vi "New_DetectionElectrodes.vi"() -> (2 "AreaName":string)   [LabVIEW 2014, in "DetectElectros.lvlib"]
uses:
  DetectElectros.lvlib
  <vilib>/Utility/file.llb/Read From Spreadsheet File (string).vi
  DataBase/DataBase.lvlib
panel:
  in  "导入电极s":path caption="导入数据"
  out "数组":string[](array[string])
  in  "OK":bool
  in  "退出":bool
  in  "提交数据":bool
  in  "导入电极":bool
  in  "电极管理_新增":string[][](table)
  in  "电极管理_新增列表":i32[](listbox)
  in  "区域名称":u16(ring) items=["1区", "2区"]
  out "error out":errorcluster caption="错误输出"
  in  "error in (no error)":errorcluster caption="错误输入（无错误）"
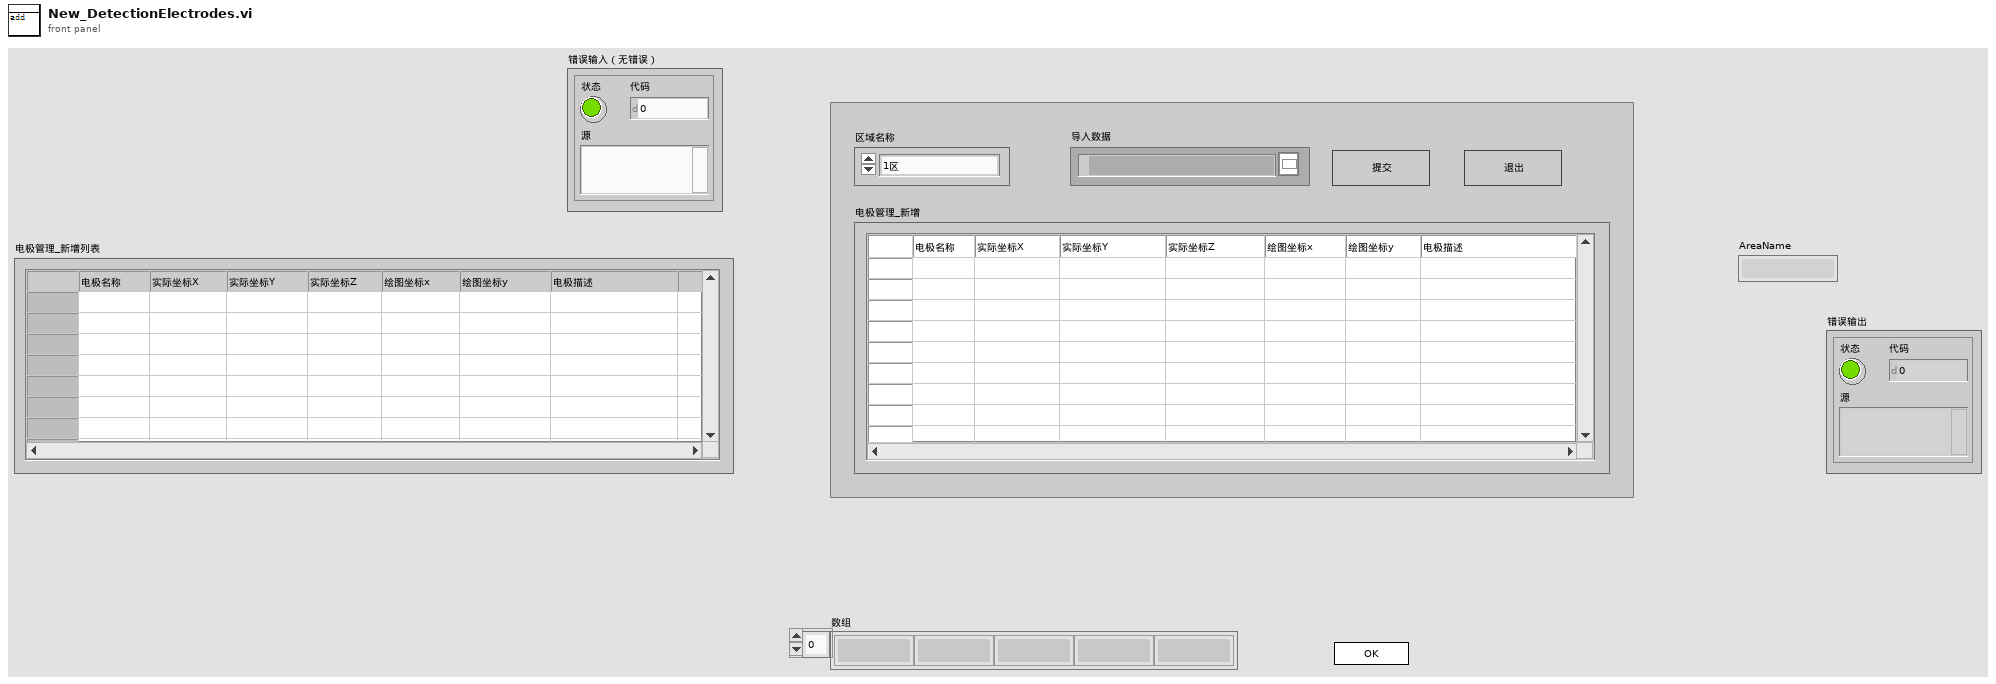
[diagram p1: front panel]
types:
  T1 = enum32{"invalid app kind", "Development System", "Run Time System", "Student Edition", "Embedded LabVIEW", "Evaluation", "Custom"}
  T2 = enum32{"Invalid", "Standard", "Closed", "Hidden", "Minimized", "Maximized"}
  T3 = cluster{"Core":cluster{"Current VI Reference":refnum<vi>, "Close Panel on Exit?":bool}, "Your Boolean data":bool, "Your string data":string, "AreaNameD":string}
  T4 = cluster{"Current VI Reference":refnum<vi>, "Close Panel on Exit?":bool}
  T5 = cluster{"String":string, "String":string, "String":string, "String":string, "String":string, "String":string, "String":string, "String":string, "String":string, "String":string, "String":string, "String":string}
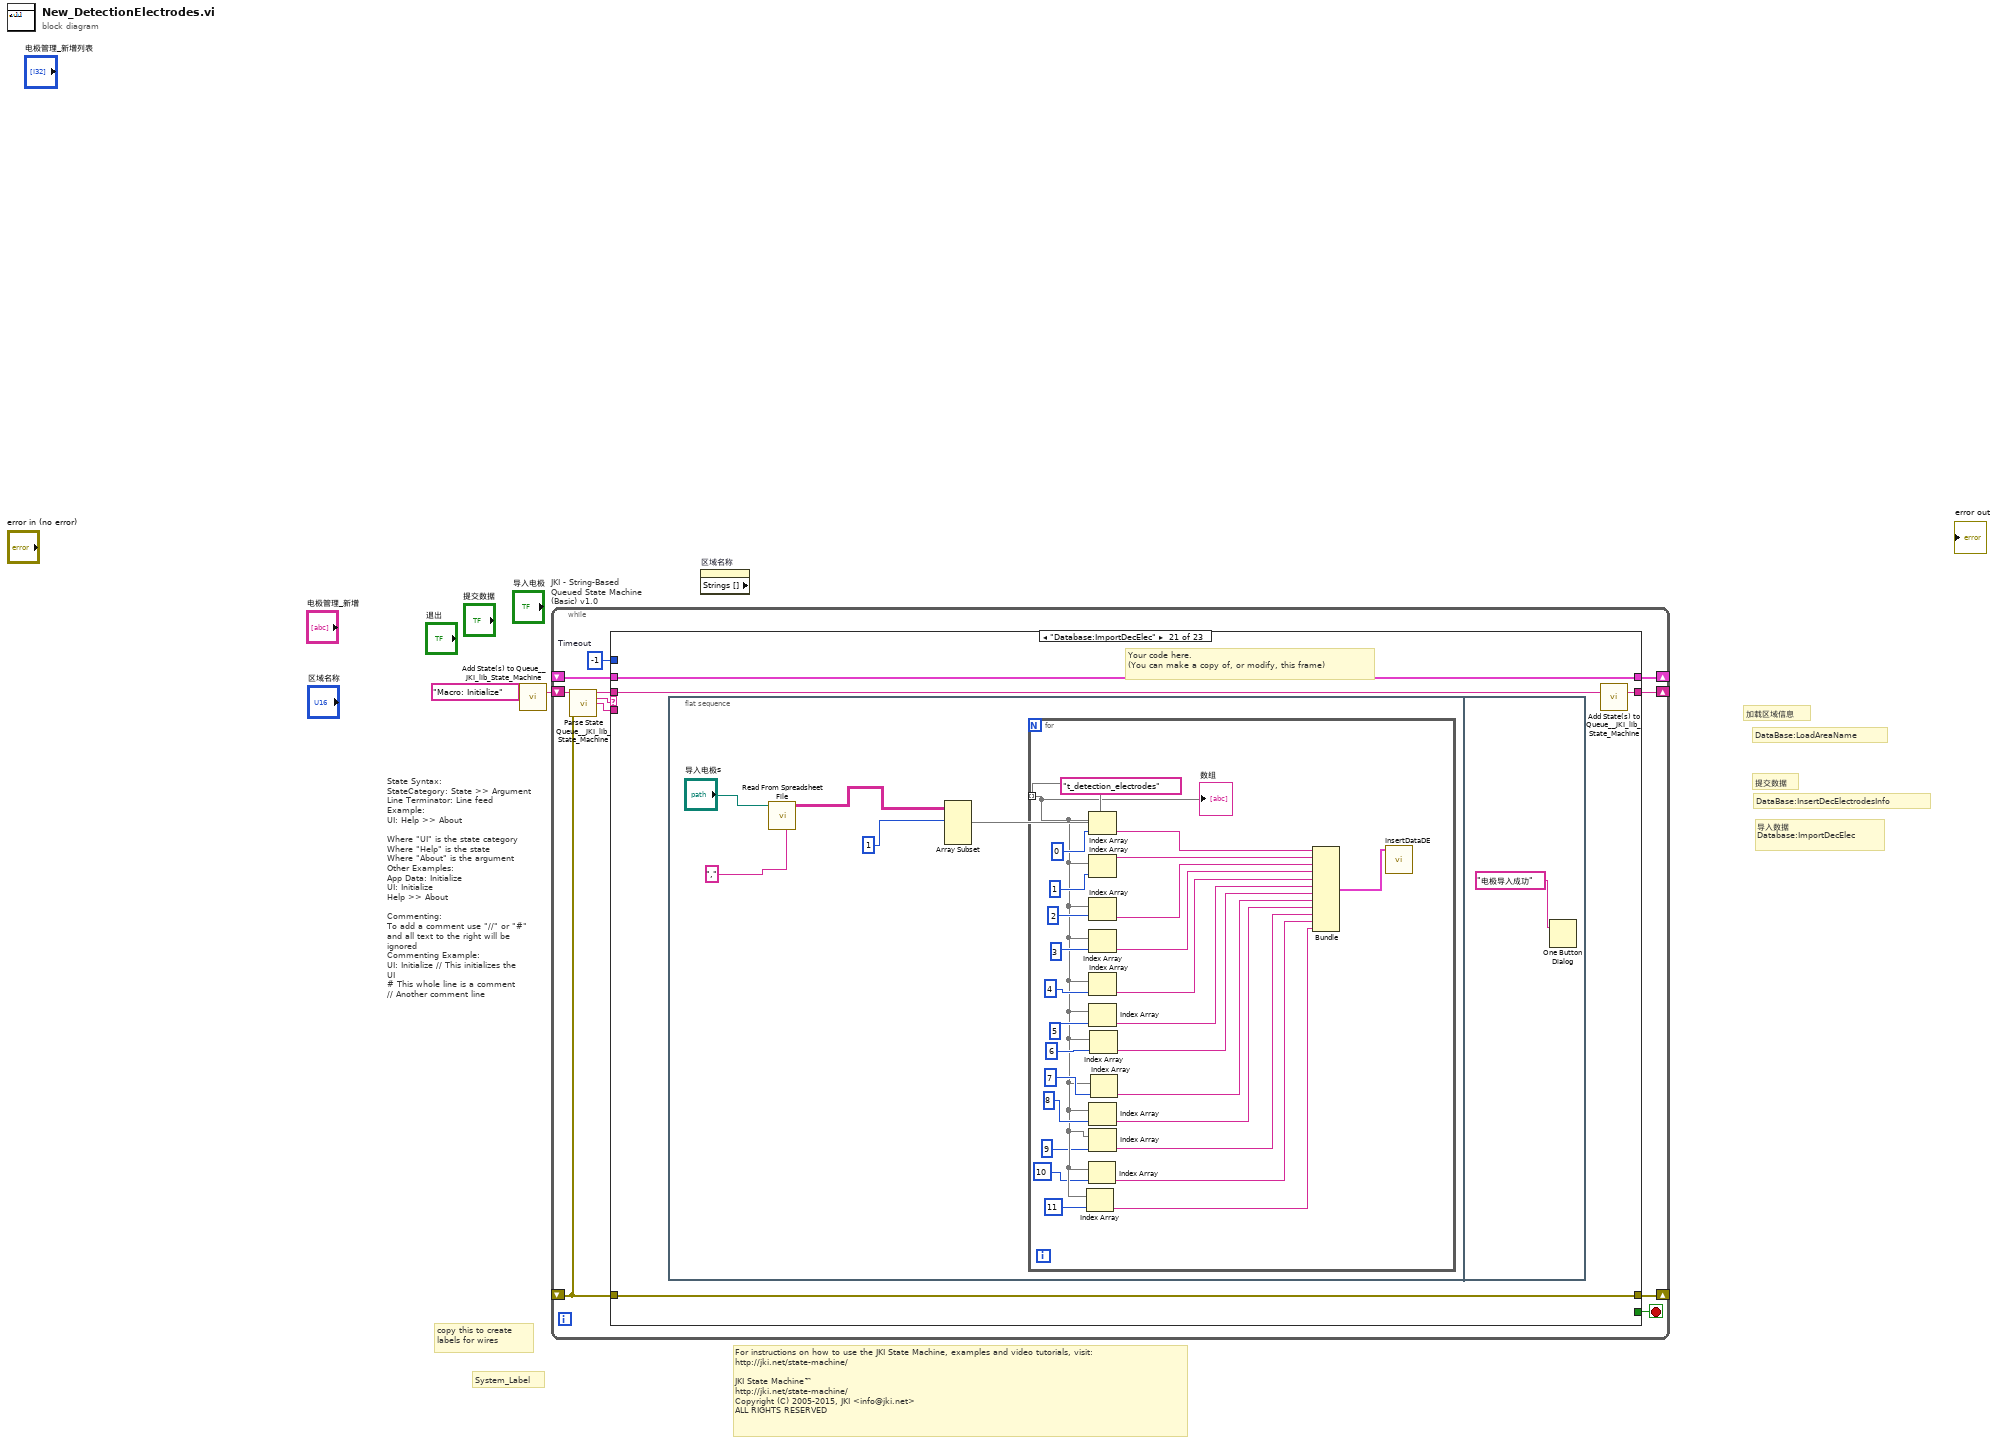
[diagram p0: block diagram]
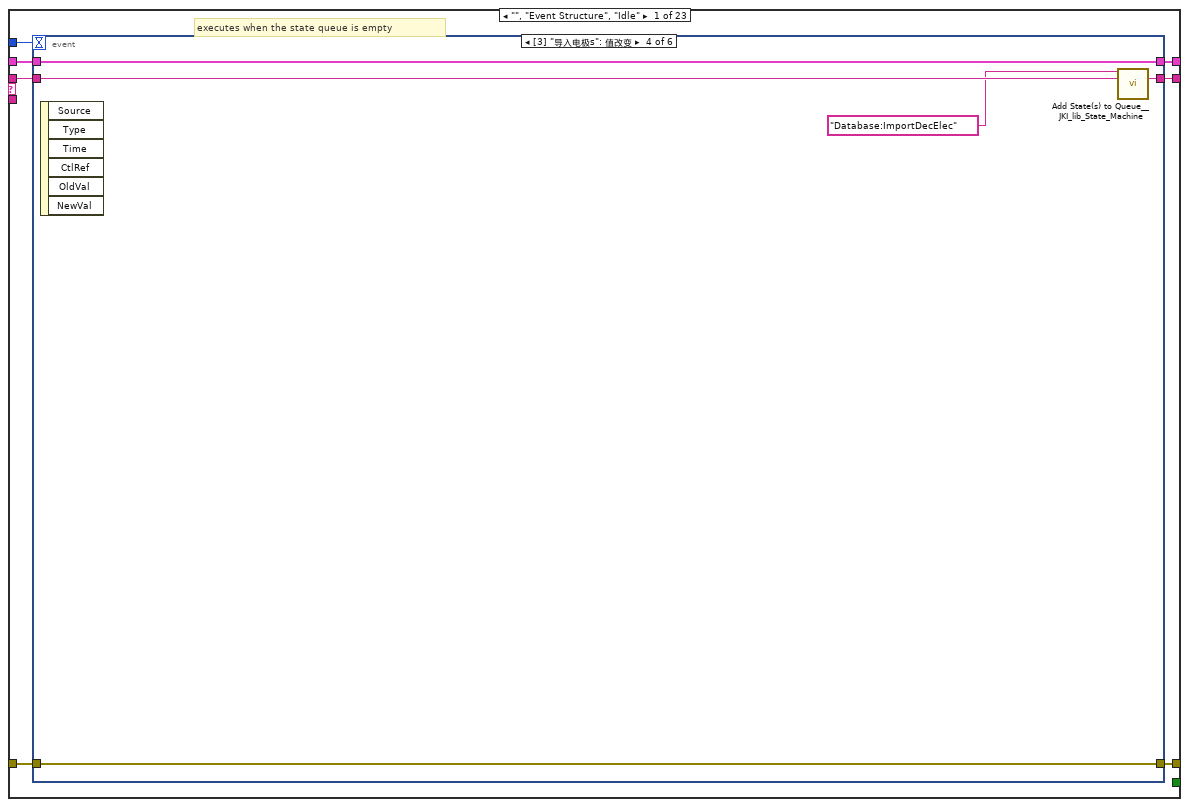
[diagram p2: hidden frame]
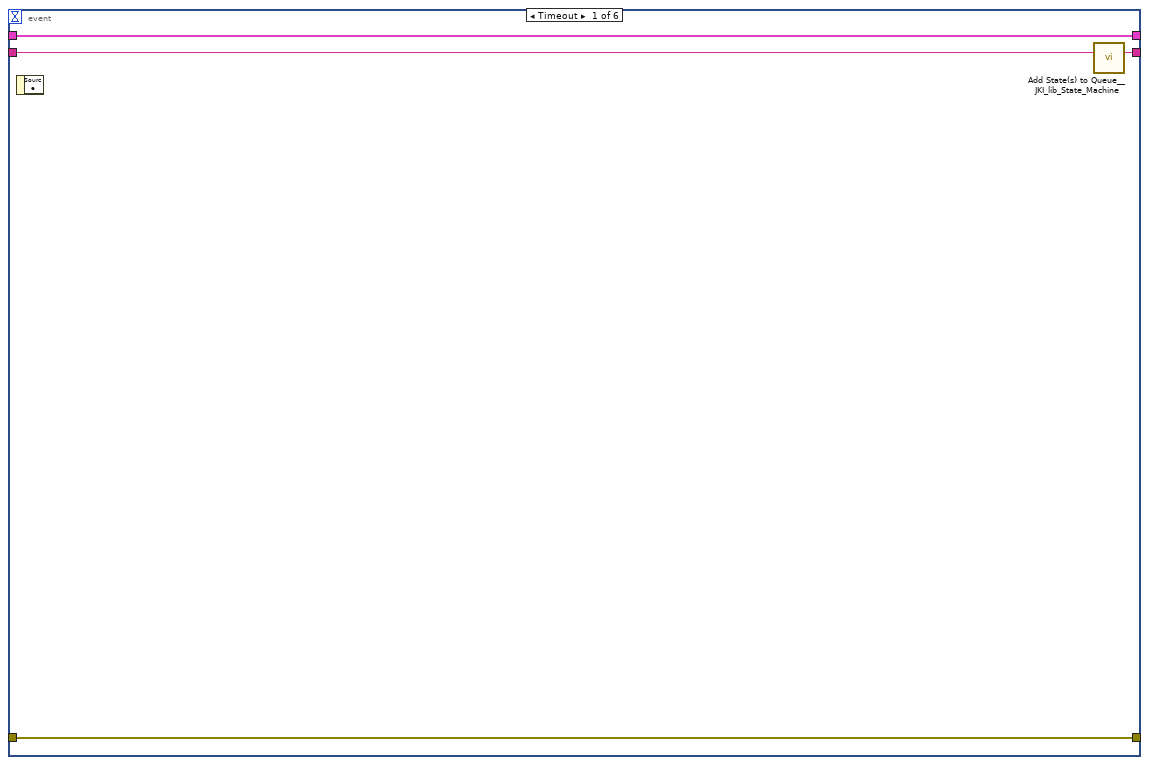
[diagram p3: hidden frame]
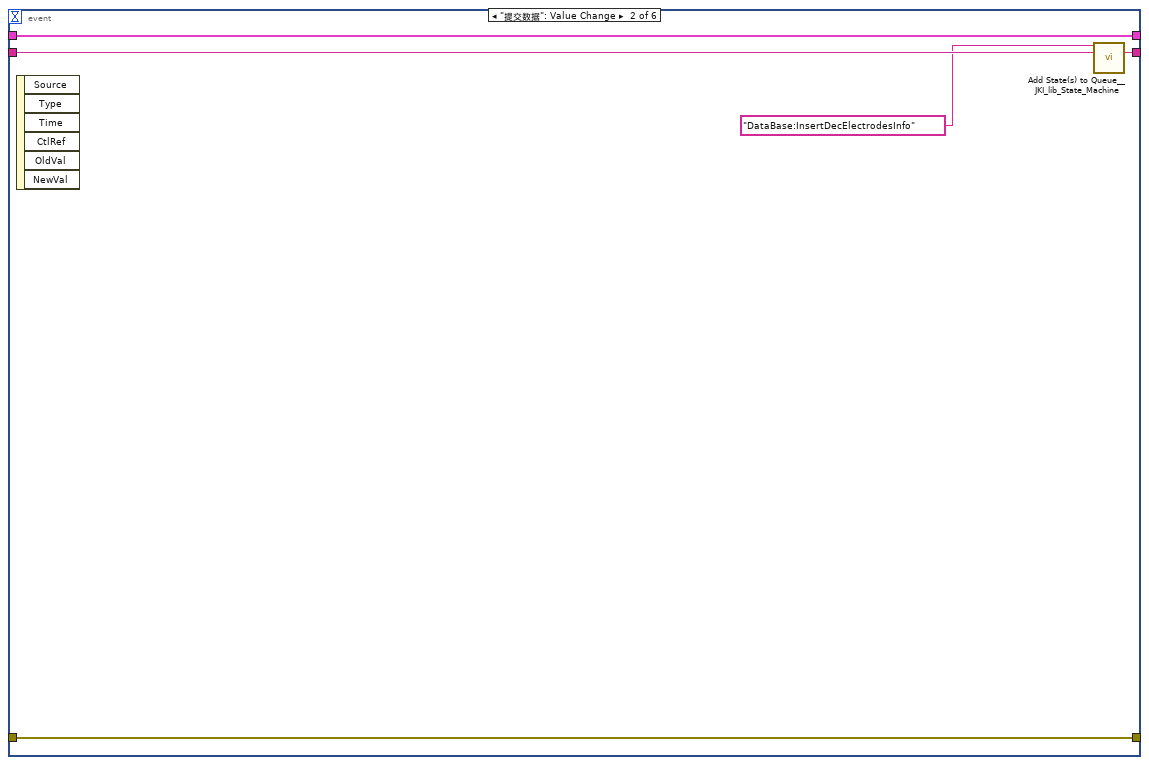
[diagram p4: hidden frame]
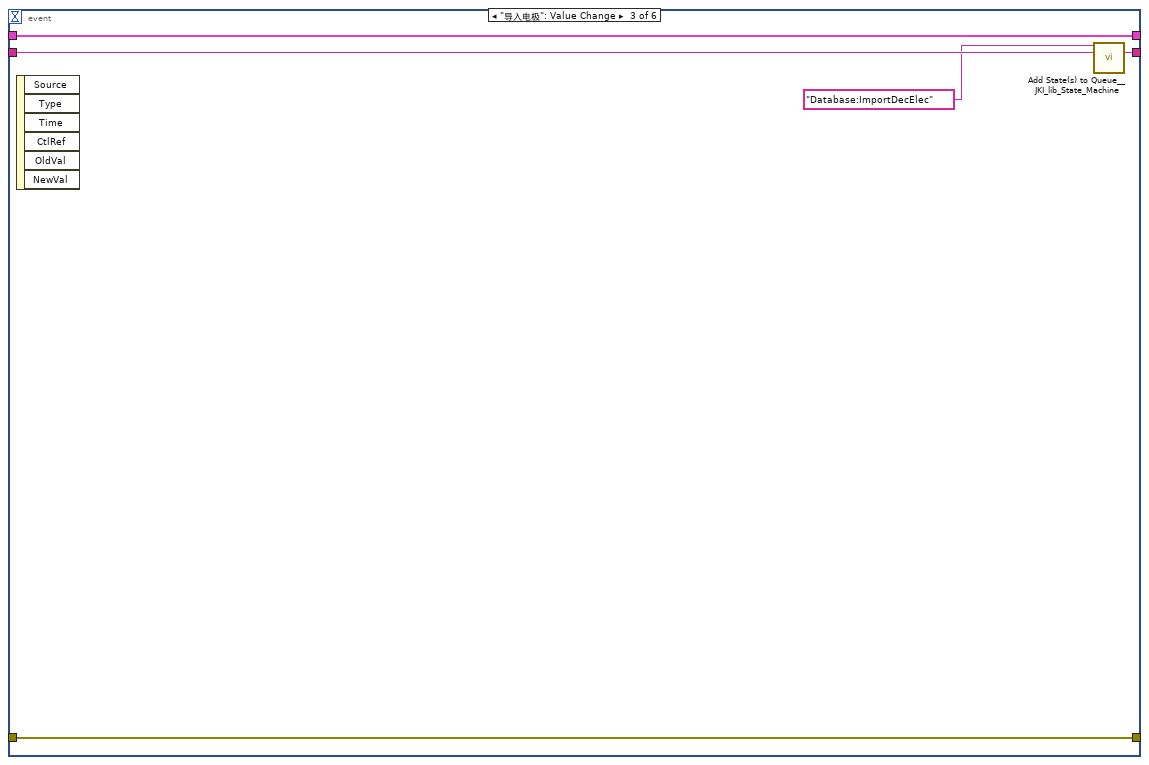
[diagram p5: hidden frame]
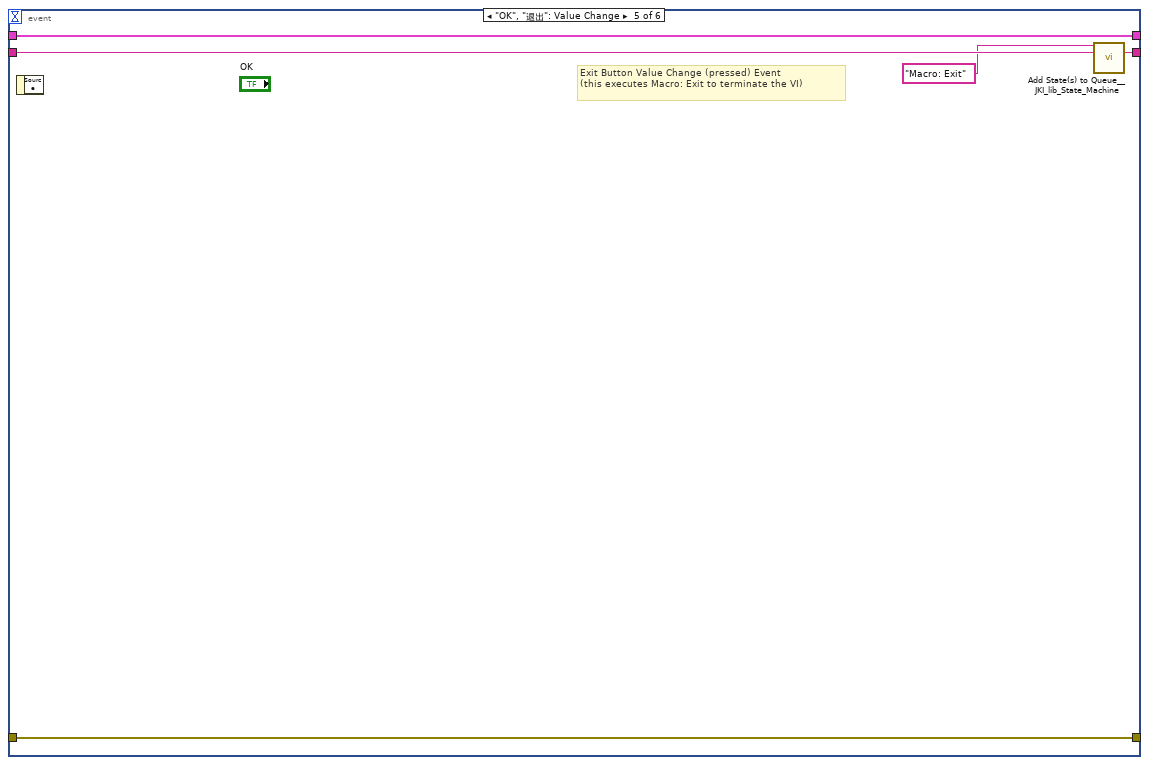
[diagram p6: hidden frame]
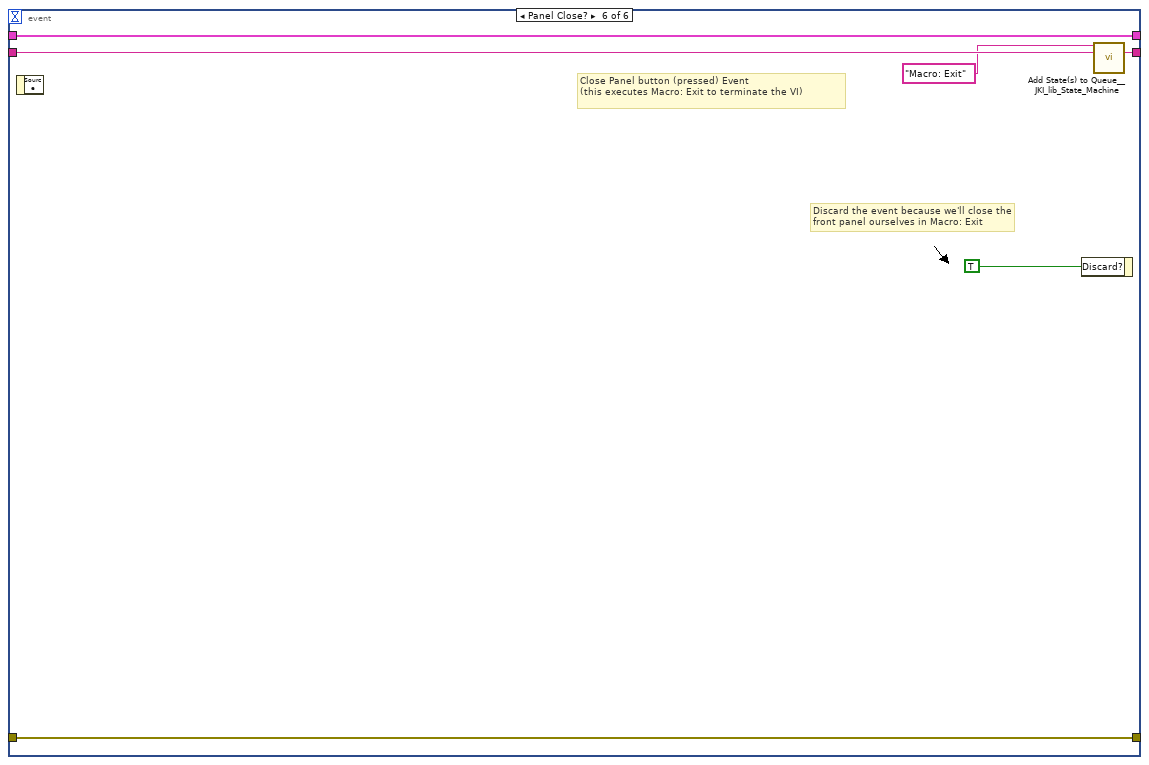
[diagram p7: hidden frame]
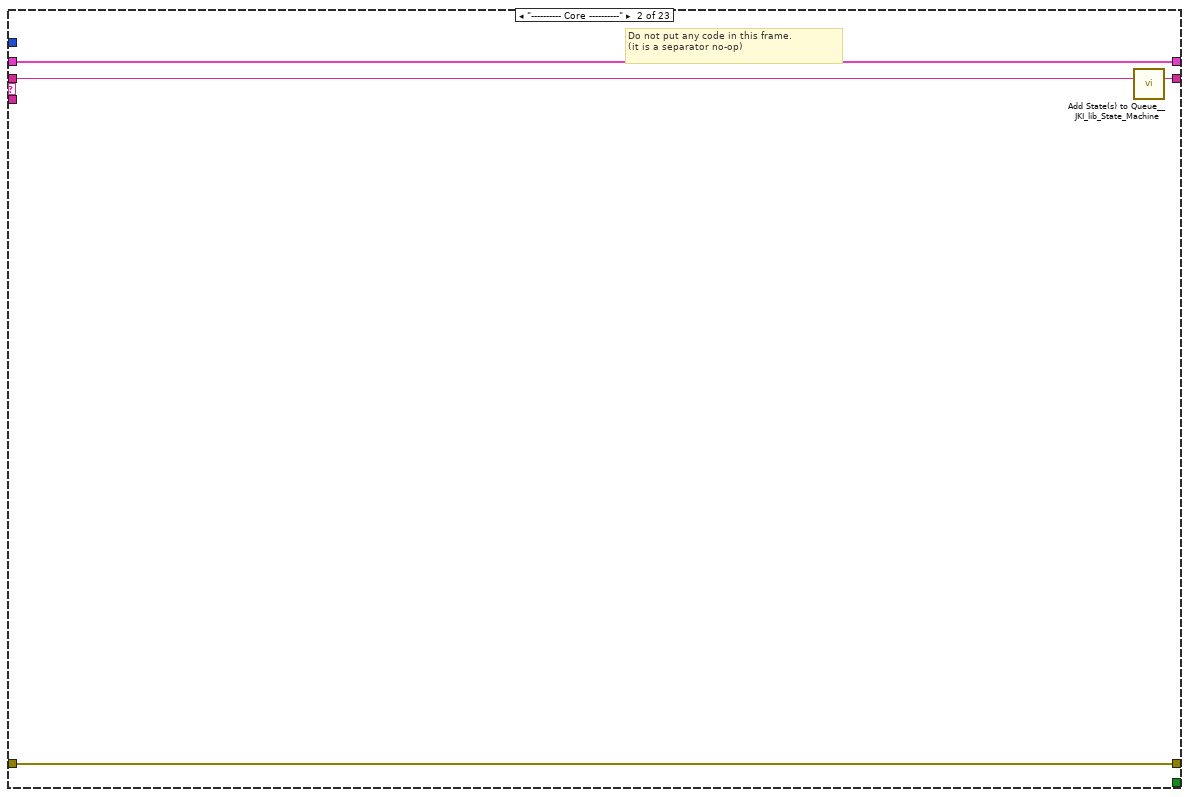
[diagram p8: hidden frame]
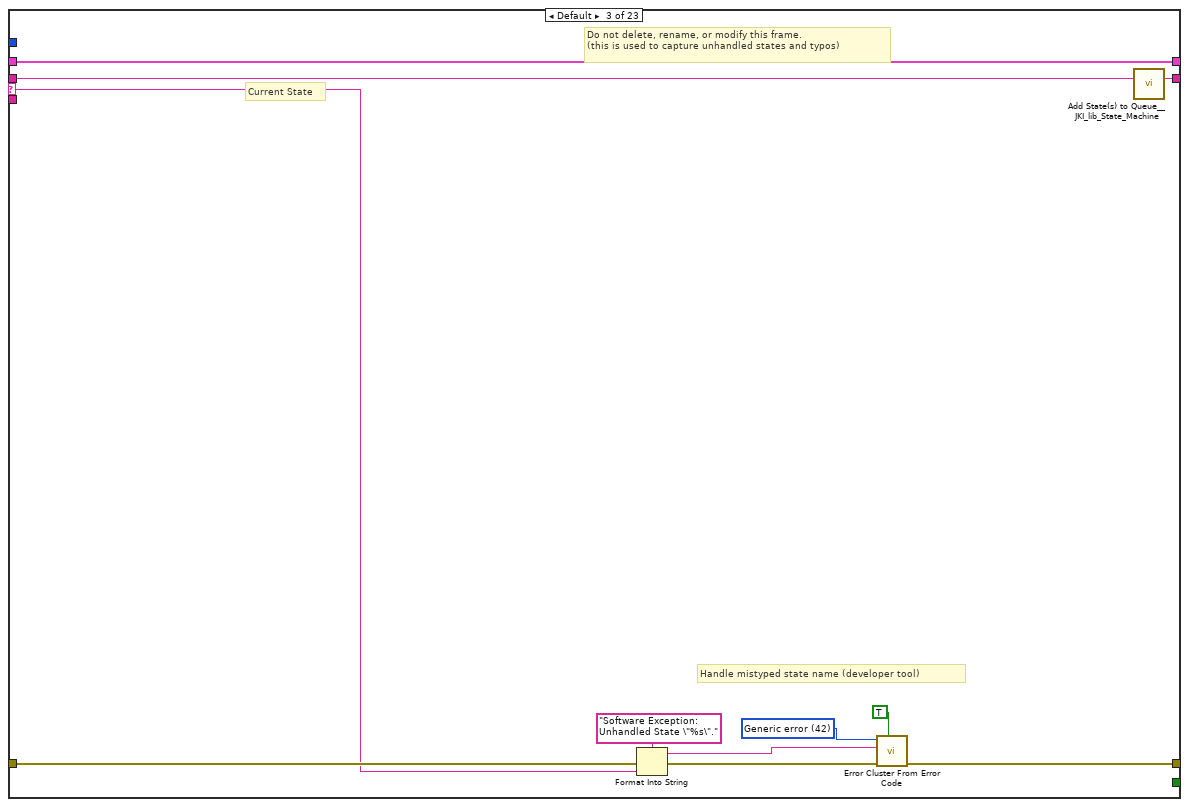
[diagram p9: hidden frame]
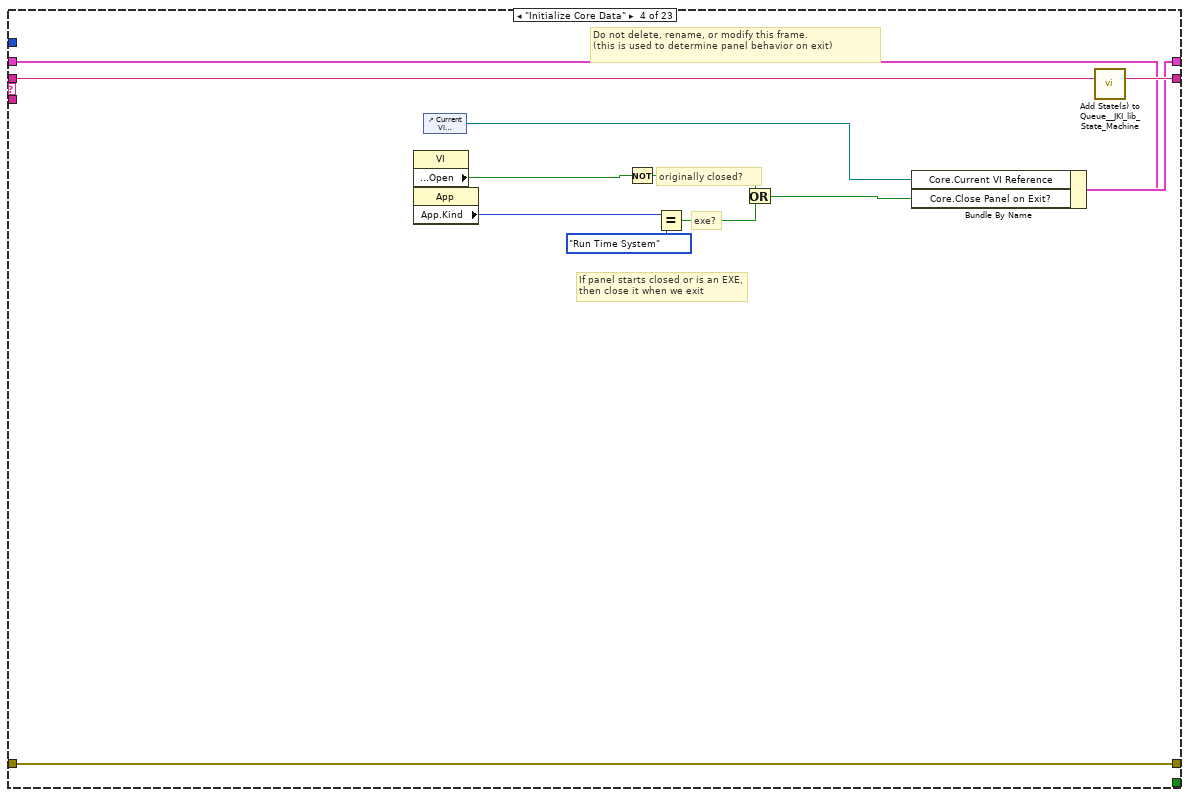
[diagram p10: hidden frame]
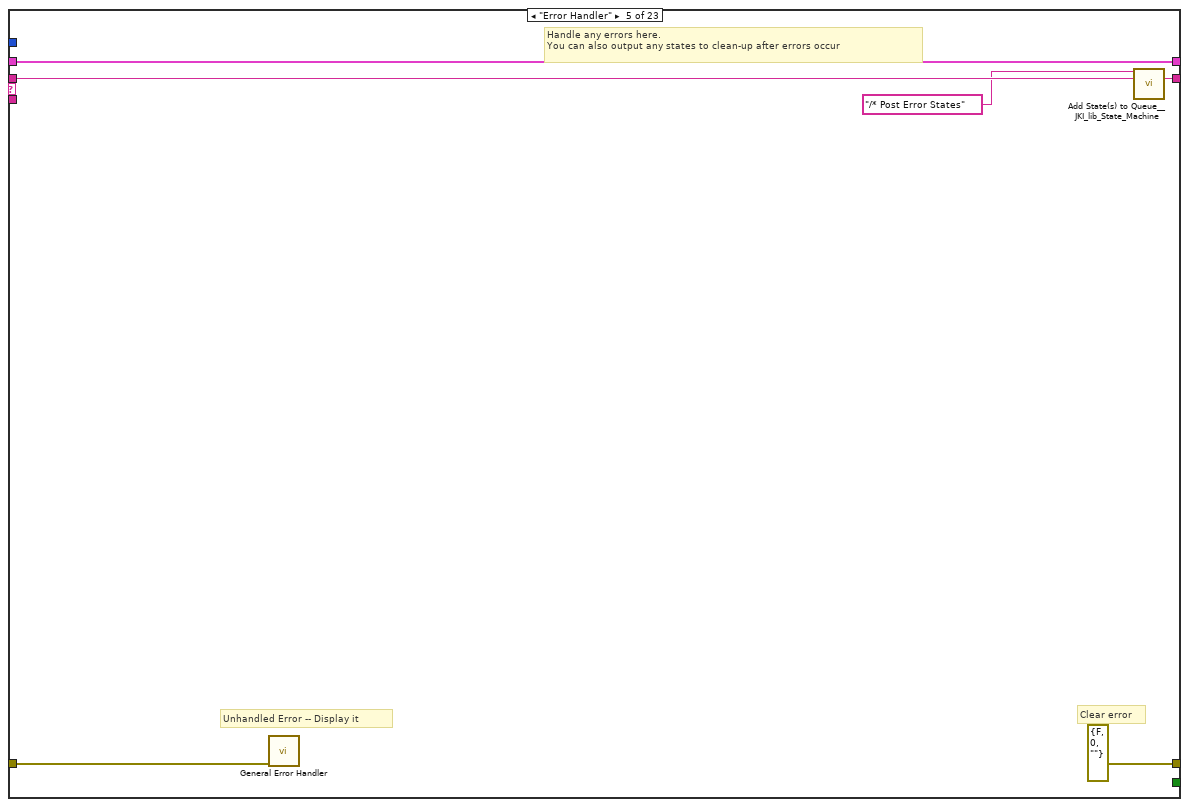
[diagram p11: hidden frame]
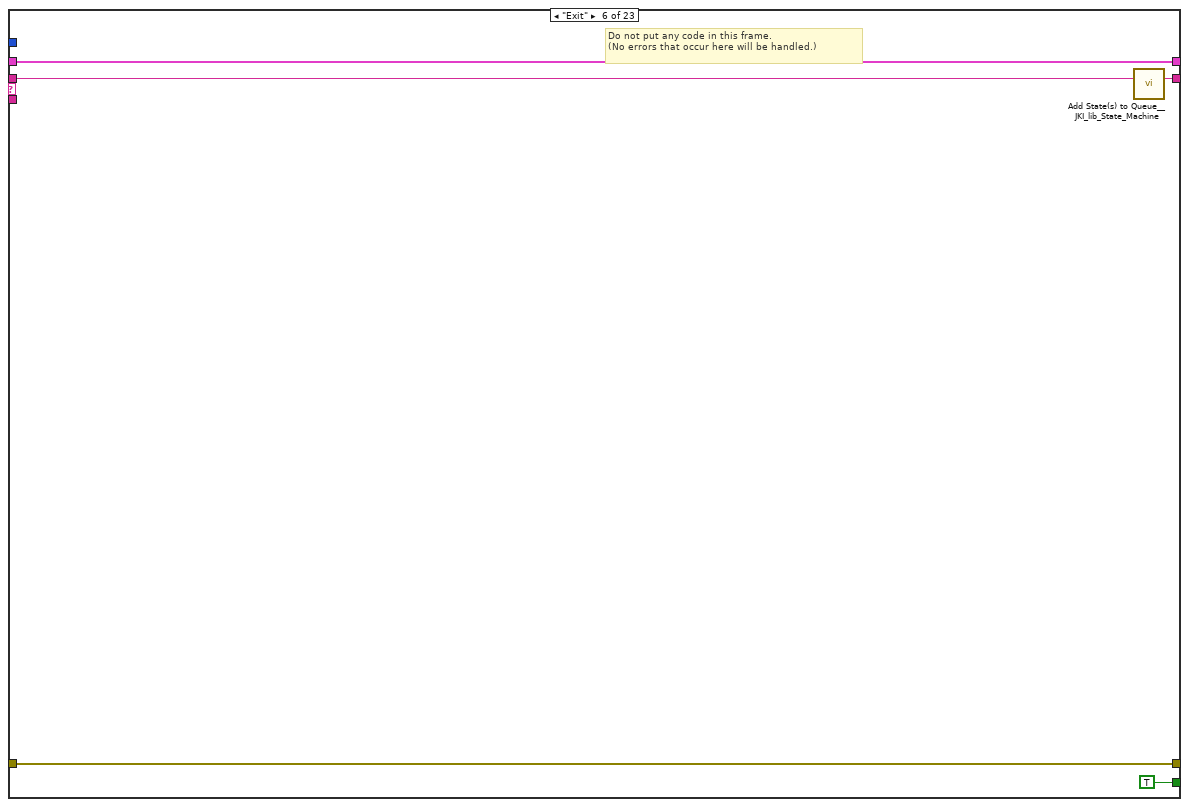
[diagram p12: hidden frame]
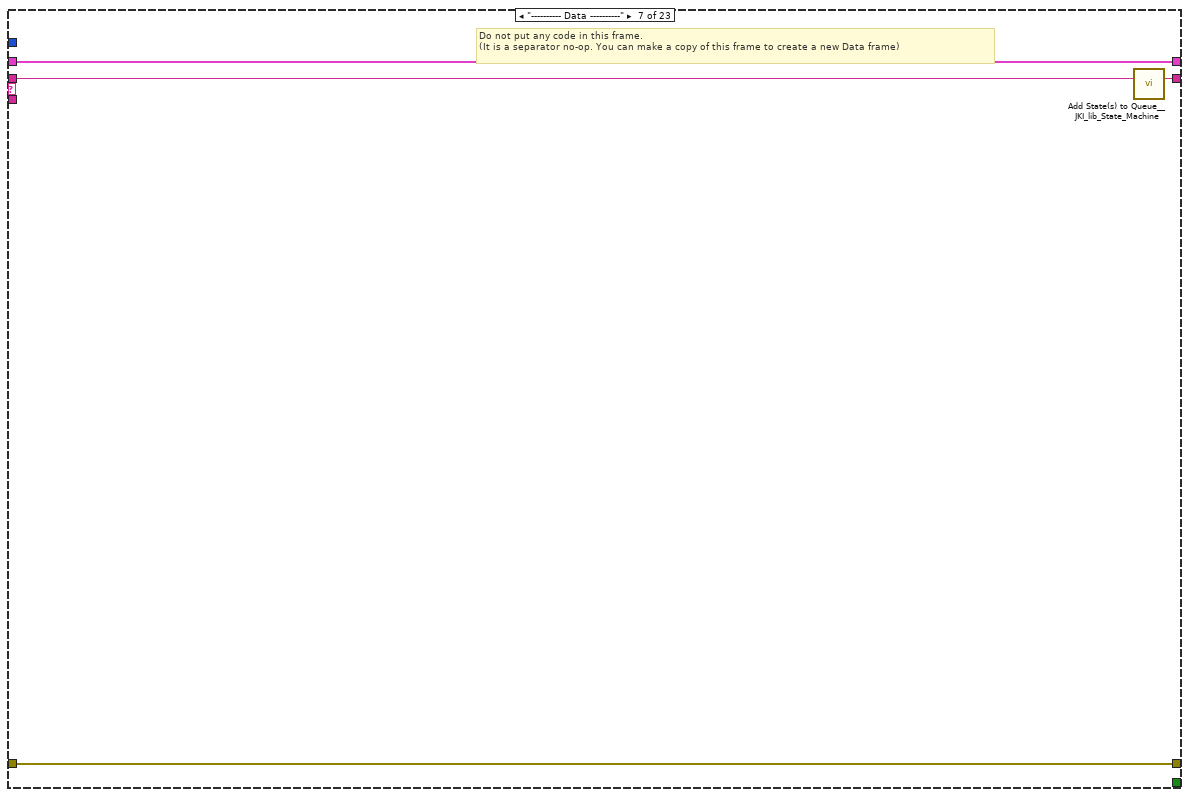
[diagram p13: hidden frame]
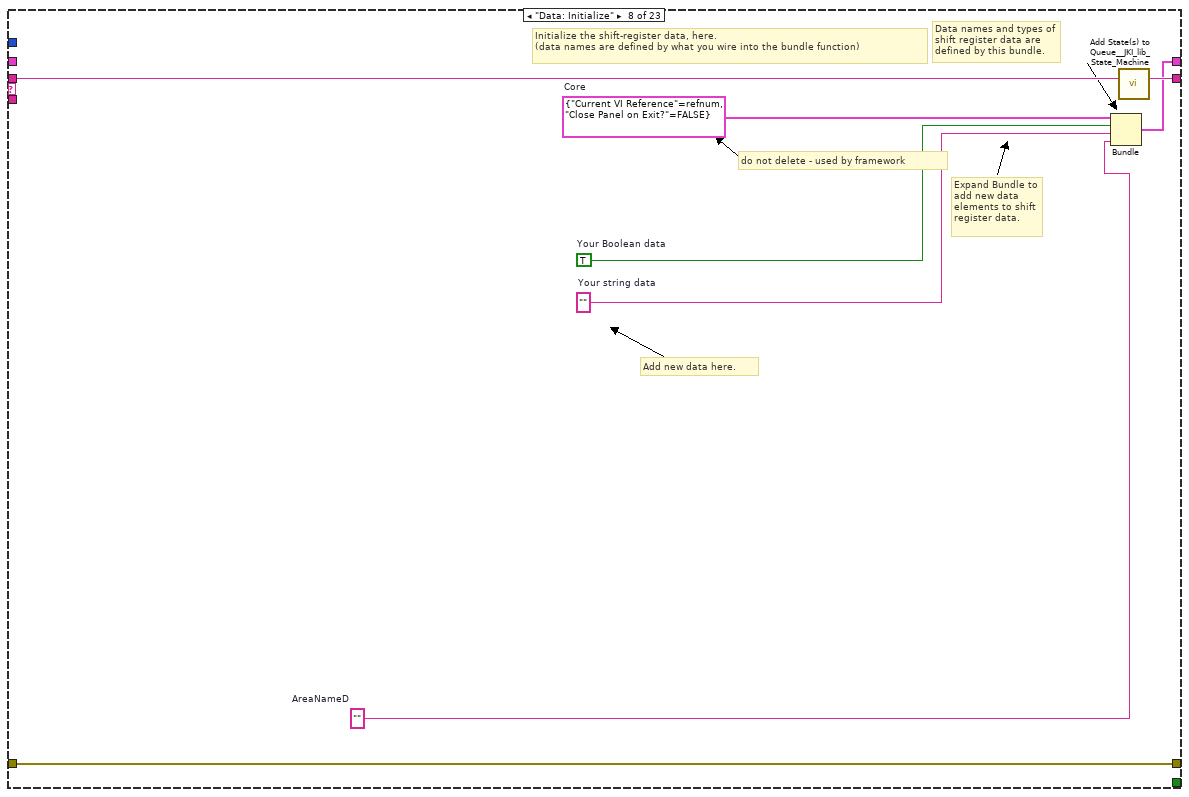
[diagram p14: hidden frame]
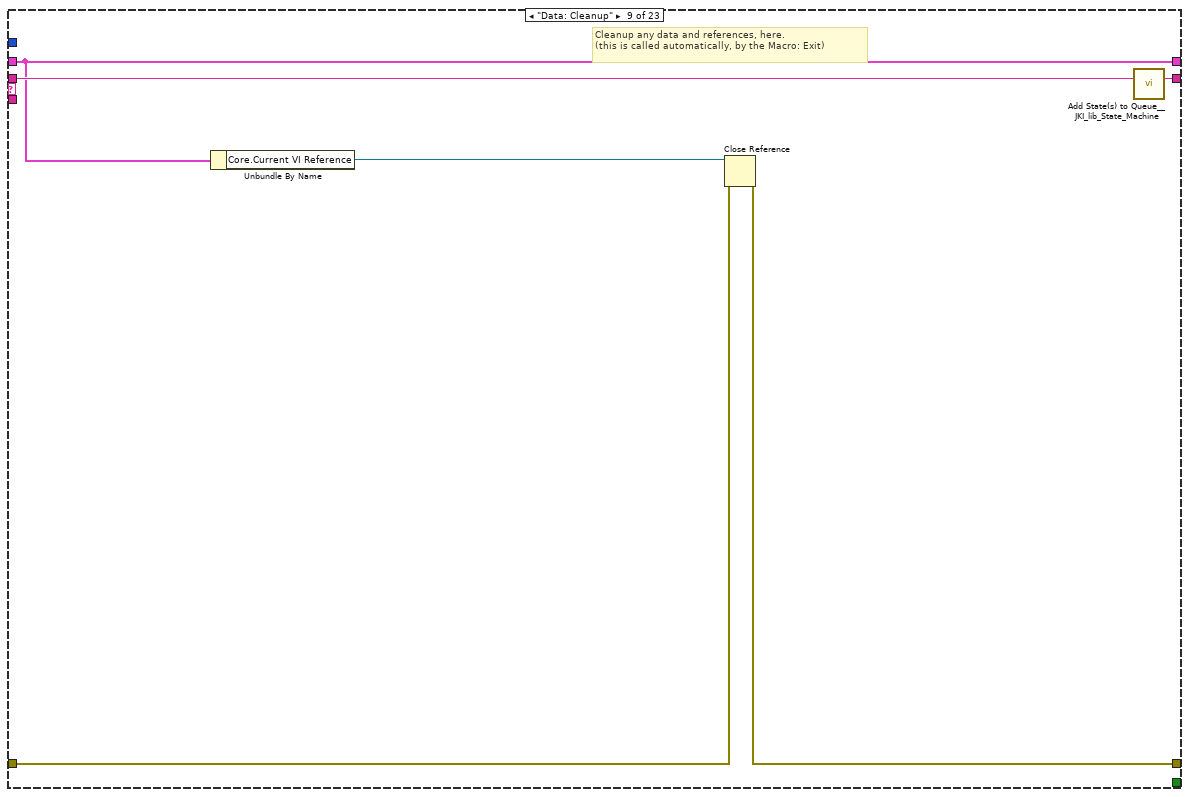
[diagram p15: hidden frame]
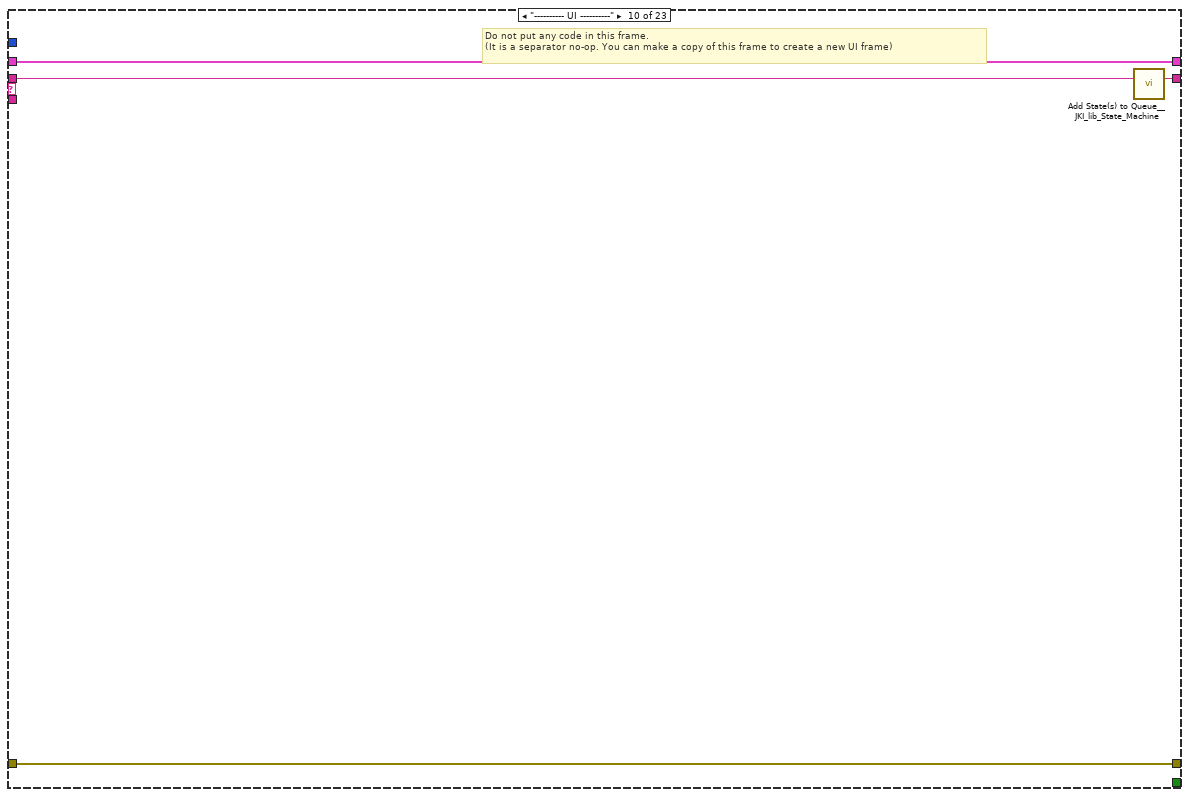
[diagram p16: hidden frame]
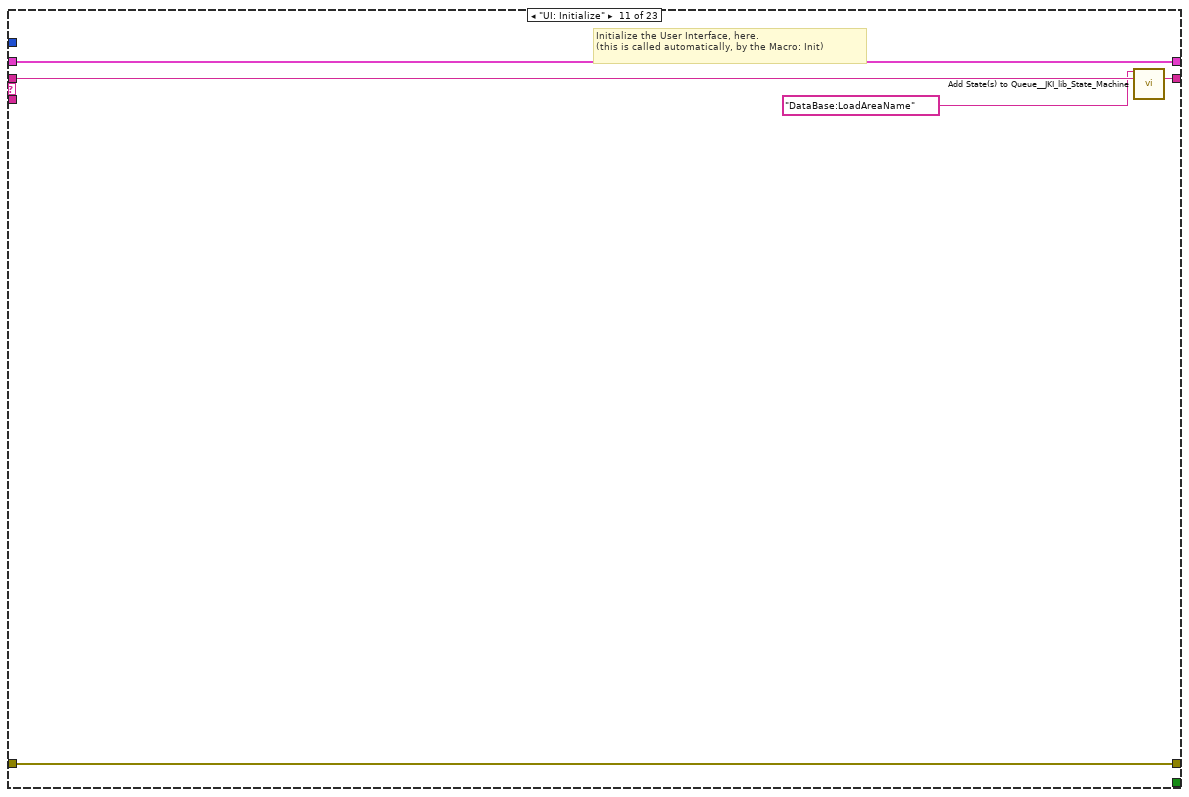
[diagram p17: hidden frame]
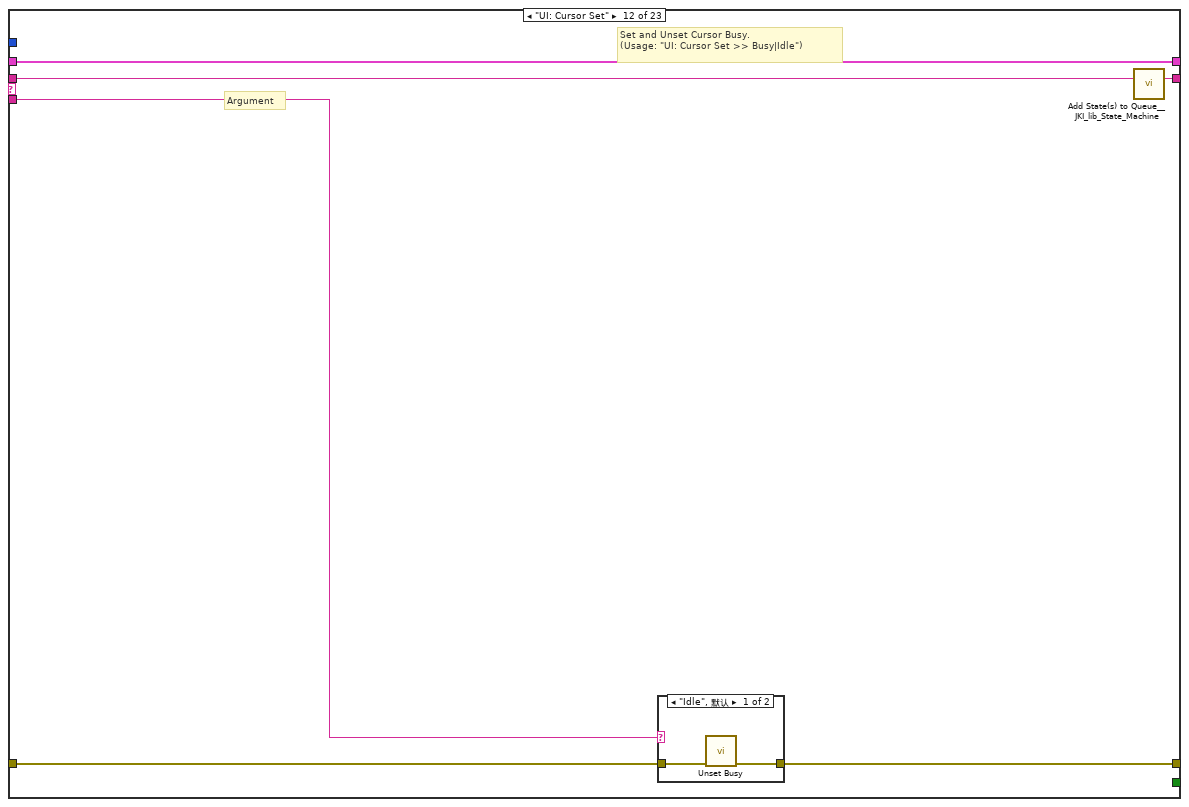
[diagram p18: hidden frame]
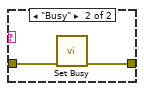
[diagram p19: hidden frame]
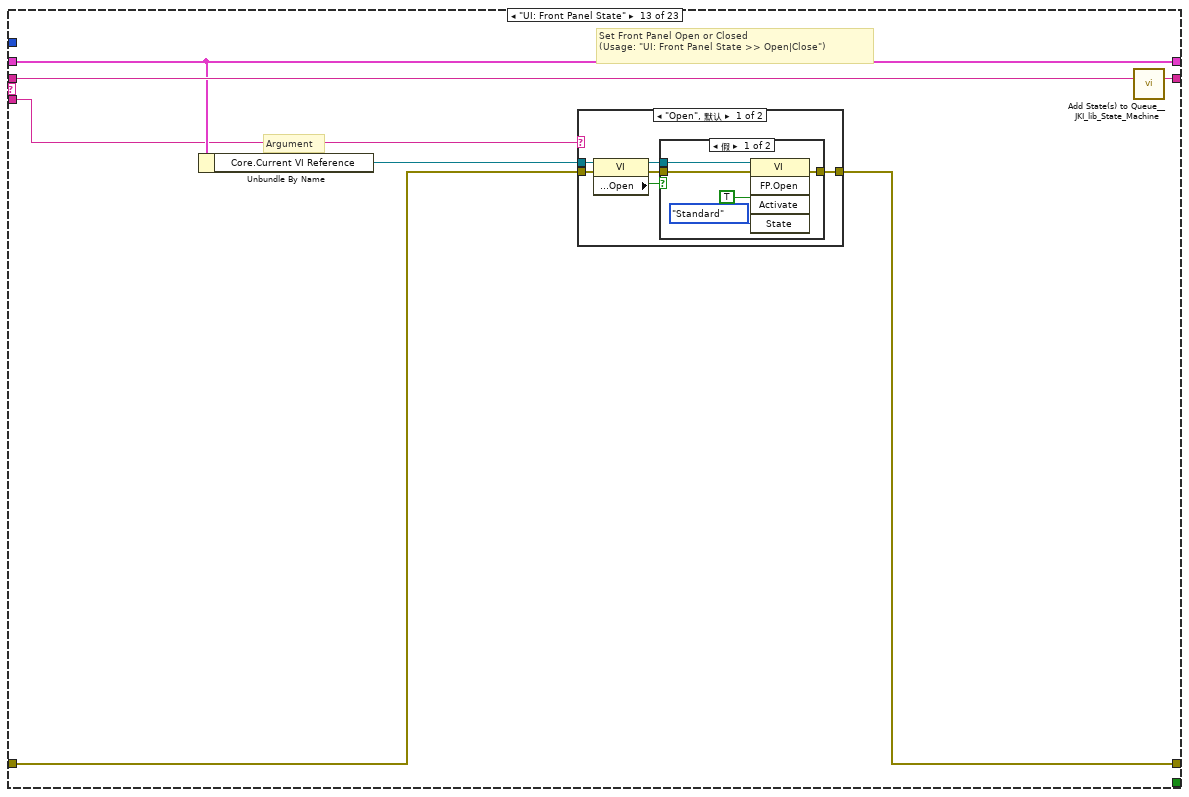
[diagram p20: hidden frame]
diagram:
  # "导入数据\nDatabase:ImportDecElec"
  # "DataBase:InsertDecElectrodesInfo"
  # "提交数据"
  # "DataBase:LoadAreaName"
  # "加载区域信息"
  # "For instructions on how to use the JKI State Machine, examples and video tutorials, visit:\nhttp://jki.net/state-machine/\n\nJKI State Machine™\nhttp://jki.net/state-machine/\nCopyright (C) 2005-2015, JKI <info@jki.net>\nALL RIGHTS RESERVED"
  # "State Syntax:\nStateCategory: State >> Argument\nLine Terminator: Line feed\nExample:\nUI: Help >> About\n\nWhere \"UI\" is the state category\nWhere \"Help\" is the state\nWhere \"About\" is the argument\nOther Examples:\nApp Data: Initialize\nUI: Initialize\nHelp >> About\n\nCommenting:\nTo add a comment use \"//\" or \"#\" and all text to the right will be ignored\nCommenting Example:\nUI: Initialize // This initializes the UI\n# This whole line is a comment\n// Another comment line"
  # "copy this to create labels for wires"
  # "System_Label"
  n1 = call <vilib>:"Add State(s) to Queue__JKI_lib_State_Machine.vi"("State(s) in (\"\")"="Macro: Initialize") -> ("States Out"=w2:string)  [unwired: 14 in]
  n2 = while "JKI - String-Based Queued State Machine (Basic) v1.0" {
    shift-right: [w6] -> _
    shift-left: _ -> [w5]
    shift-right: [w9] -> _
    shift-left: _ -> [w3]
    shift-right: [w8] -> _
    shift-left: w2 -> [w10]
    stop <- w7 stop-if-true
    w4 = -1  # Timeout
    n3 = call <vilib>:"Parse State Queue__JKI_lib_State_Machine.vi"("State Queue"=w10, "Error In (no error)"=w3) -> ("Remaining States"=w12:string, "Current State"=w13:string, "Arguments"=w11:string)  [unwired: 11 in]
    n4 = case shown="\"Database:ImportDecElec\"" w13 {
      selector: w13 -> [_ _ w55 _ _ _ _ _ _ _ _ _ _ _ _ _ _ _ _ _ _ _ _]
      tunnel: w12 -> [w20 w54 w59 w77 w83 w88 w92 w100 w106 w110 w115 w121 w132 w158 w163 w173 w177 w181 w185 w189 w193 w233 w259]
      tunnel: w11 -> [_ _ _ _ _ _ _ _ _ _ _ w116 w126 _ _ _ _ _ _ _ _ _ _]
      tunnel: w5 -> [w18 w51 w57 w68 w80 w86 w89 _ w101 w107 w113 w119 w128 w155 w160 w170 w174 w178 w182 w186 w190 w226 w247]
      tunnel: [w17 w52 w61 w74 errorcluster {"status"=FALSE, "code"=0, "source"=""} ("error out") w85 w90 w97 w102 w108 w112 w117 w129 w156 w161 w171 w175 w179 w183 w187 w191 w227 w251] -> w9
      tunnel: w3 -> [w16 w52 w60 w74 w79 w85 w90 w97 w103 w108 w112 w118 w130 w156 w161 w171 w175 w179 w183 w187 w191 w228 w251]
      tunnel: [w19 w53 w58 w76 w82 w87 w91 w99 w105 w109 w114 w120 w131 w157 w162 w172 w176 w180 w184 w188 w192 w232 w258] -> w8
      tunnel: [_ _ _ _ _ TRUE _ _ _ _ _ _ _ _ _ _ _ _ _ _ _ _ _] -> w7
      tunnel: [w15 w51 w57 w75 w80 w86 w89 w98 w101 w107 w113 w119 w128 w155 w160 w170 w174 w178 w182 w186 w190 w226 w246] -> w6
      tunnel: w4 -> [w14 _ _ _ _ _ _ _ _ _ _ _ _ _ _ _ _ _ _ _ _ _ _]
      frame "", "Event Structure", "Idle" {
        # "executes when the state queue is empty"
        n5 = event shown="[3] \"导入电极s\": 值改变" {
          selector: _ -> [_ _ _ _ _ _]
          dyn-events: _ -> [_ _ _ _ _ _]
          timeout: w14 -> [_ _ _ _ _ _]
          tunnel: w20 -> [w24 w29 w34 w39 w44 w50]
          tunnel: [w23 w28 w33 w38 w43 w49] -> w19
          tunnel: w18 -> [w21 w26 w31 w36 w41 w47]
          tunnel: [w22 w27 w32 w37 w42 w48] -> w17
          tunnel: w16 -> [w22 w27 w32 w37 w42 w48]
          tunnel: [w21 w26 w31 w36 w41 w47] -> w15
          event Timeout {
            n6 = event-data() -> ()  [unwired: 1 in, 1 out]
            n7 = call <vilib>:"Add State(s) to Queue__JKI_lib_State_Machine.vi"("State(s) in (\"\")"=w24) -> ("States Out"=w23:string)  [unwired: 14 in]
          }
          event "提交数据": Value Change {
            n8 = event-data() -> ()  [unwired: 1 in, 6 out]
            n9 = call <vilib>:"Add State(s) to Queue__JKI_lib_State_Machine.vi"("State(s) in Front (\"\")"="DataBase:InsertDecElectrodesInfo", "State(s) in (\"\")"=w29) -> ("States Out"=w28:string)  [unwired: 13 in]
          }
          event "导入电极": Value Change {
            n10 = event-data() -> ()  [unwired: 1 in, 6 out]
            n11 = call <vilib>:"Add State(s) to Queue__JKI_lib_State_Machine.vi"("State(s) in Front (\"\")"="Database:ImportDecElec", "State(s) in (\"\")"=w34) -> ("States Out"=w33:string)  [unwired: 13 in]
          }
          event "导入电极s": Value Change {
            n12 = event-data() -> ()  [unwired: 1 in, 6 out]
            n13 = call <vilib>:"Add State(s) to Queue__JKI_lib_State_Machine.vi"("State(s) in Front (\"\")"="Database:ImportDecElec", "State(s) in (\"\")"=w39) -> ("States Out"=w38:string)  [unwired: 13 in]
          }
          event "OK", "退出": Value Change {
            # "Exit Button Value Change (pressed) Event\n(this executes Macro: Exit to terminate the VI)"
            n14 = event-data() -> ()  [unwired: 1 in, 1 out]
            n15 = call <vilib>:"Add State(s) to Queue__JKI_lib_State_Machine.vi"("State(s) in Front (\"\")"="Macro: Exit", "State(s) in (\"\")"=w44) -> ("States Out"=w43:string)  [unwired: 13 in]
          }
          event Panel Close? {
            # "Discard the event because we'll close the front panel ourselves in Macro: Exit"
            # "Close Panel button (pressed) Event\n(this executes Macro: Exit to terminate the VI)"
            n16 = event-data() -> ()  [unwired: 1 in, 1 out]
            n17 = event-data("Discard?"=TRUE) -> ()  [unwired: 1 in, 1 out]
            n18 = call <vilib>:"Add State(s) to Queue__JKI_lib_State_Machine.vi"("State(s) in Front (\"\")"="Macro: Exit", "State(s) in (\"\")"=w50) -> ("States Out"=w49:string)  [unwired: 13 in]
          }
        }
      }
      frame "---------- Core ----------" {
        # "Do not put any code in this frame.\n(it is a separator no-op)"
        n19 = call <vilib>:"Add State(s) to Queue__JKI_lib_State_Machine.vi"("State(s) in (\"\")"=w54) -> ("States Out"=w53:string)  [unwired: 14 in]
      }
      frame Default {
        w64 = 42 items=["No error", "Argument error", "Memory is full", "Out of zone", "End of file", "File already open", "Generic file I/O error", "File not found", "File permission error", "Disk is full", "Duplicate path", "Too many files open", "System feature not enabled", "Resource file not found", "Cannot add resource", "Resource not found", "Image not found", "Image memory error", "Pen does not exist", "Config type invalid", "Config token not found", "Config parse error", "Config memory error", "Bad external code format", "Bad external code offset", "External code not present", "Null window", "Destroy window error", "Null menu", "Print aborted", "Bad print record", "Print driver error", "Windows error during printing", "Memory error during printing", "Print dialog error", "Generic print error", "Invalid device refnum", "Device not found", "Device parameter error", "Device unit error", "Cannot open device", "Device call aborted", "Generic error", "Cancelled by user", "Object ID too low", "Object ID too high", "Object not in heap", "Unknown heap", "Unknown object (invalid DefProc)", "Unknown object (DefProc not in table)", "Message out of range", "Invalid (null) method", "Unknown message", "Manager call not supported", "Bad address", "Network operation in progress", "Network operation timed out", "Connection is busy", "Network attribute not supported", "Network error", "Address in use", "System out of memory", "Connection aborted", "Connection refused", "Not connected", "Already connected", "Connection closed", "Initialization error (interapplication manager)", "Bad occurrence", "Wait on unbound occurrence handler", "Occurrence queue overflow", "Datalog type conflict", "Unused", "Unrecognized type (interapplication manager)", "Memory corrupt", "Failed to make temporary DLL", "Old CIN version", "Drag socket not found", "Failed to load drop-object", "Failed to register OLE object", "Failed to release OLE object", "Format specifier type mismatch", "Unknown format specifier", "Too few format specifiers", "Too many format specifiers", "Scan failed", "Newer CIN version", "Error converting to variant", "Runtime menu error", "Password tampered", "Variant attribute not found", "Incompatible variant data type", "Event data is not available", "Event Store is not present", "Occurrence is not found", "Event Queue is not created", "Event info is not available", "Refnum passed is NULL", "Error retrieving Class GUID", "Error retrieving CoClass GUID", "Error retrieving TypeLib GUID.", "Bad built application magic bytes.", "Specific driver is different from the specific driver associated with the Logical Name.", "There is no session opened to the class driver.", "Max Error", "MAX - Error with config objects", "MAX - Error loading configuration", "MAX - Group not supported"]
        # "Current State"
        # "Do not delete, rename, or modify this frame.\n(this is used to capture unhandled states and typos)"
        # "Handle mistyped state name (developer tool)"
        n20 = Format Into String(format string="Software Exception: Unhandled State \"%s\"." ("message"), error in=w60, w55) -> (resulting string=w63:string, error out=w62:errorcluster)  [unwired: 1 in]
        n21 = call <vilib>:"Error Cluster From Error Code.vi"("show call chain? (False)"=TRUE, "error in (no error)"=w62, "error message (\"\")"=w63, "error code (0)"=w64) -> ("error out"=w61:errorcluster)  [unwired: 5 in]
        n22 = call <vilib>:"Add State(s) to Queue__JKI_lib_State_Machine.vi"("State(s) in (\"\")"=w59) -> ("States Out"=w58:string)  [unwired: 14 in]
      }
      frame "Initialize Core Data" {
        # "Do not delete, rename, or modify this frame.\n(this is used to determine panel behavior on exit)"
        # "originally closed?"
        # "exe?"
        # "If panel starts closed or is an EXE, then close it when we exit"
        n23 = property class="VI"() -> ("Front Panel.Open"=w73:bool)  [unwired: 2 in, 2 out]
        n24 = property class="App"() -> ("App.Kind"=w72:T1)  [unwired: 2 in, 2 out]
        n25 = control-ref of="Current VI Reference"() -> (w66:refnum<vi>)
        n26 = Not(x=w73) -> (.not. x?=w70:bool)
        n27 = Equal?(x=w72, y=T1."Run Time System" ("Application:Kind")) -> (x = y?=w69:bool)
        n28 = Or(x=w70, y=w69) -> (x .or. y?=w67:bool)
        n29 = Bundle By Name(cluster=w68, "Core.Current VI Reference"=w66, "Core.Close Panel on Exit?"=w67) -> (w75:T3)
        n30 = call <vilib>:"Add State(s) to Queue__JKI_lib_State_Machine.vi"("State(s) in (\"\")"=w77) -> ("States Out"=w76:string)  [unwired: 14 in]
      }
      frame "Error Handler" {
        # "Unhandled Error -- Display it"
        # "Handle any errors here.\nYou can also output any states to clean-up after errors occur"
        # "Clear error"
        n31 = call <vilib>:"General Error Handler.vi"("error in (no error)"=w79) -> ()  [unwired: 10 in, 5 out]
        n32 = call <vilib>:"Add State(s) to Queue__JKI_lib_State_Machine.vi"("State(s) in Front (\"\")"="/* Post Error States", "State(s) in (\"\")"=w83) -> ("States Out"=w82:string)  [unwired: 13 in]
      }
      frame "Exit" {
        # "Do not put any code in this frame.\n(No errors that occur here will be handled.)"
        n33 = call <vilib>:"Add State(s) to Queue__JKI_lib_State_Machine.vi"("State(s) in (\"\")"=w88) -> ("States Out"=w87:string)  [unwired: 14 in]
      }
      frame "---------- Data ----------" {
        # "Do not put any code in this frame.\n(It is a separator no-op. You can make a copy of this frame to create a new Data frame)"
        n34 = call <vilib>:"Add State(s) to Queue__JKI_lib_State_Machine.vi"("State(s) in (\"\")"=w92) -> ("States Out"=w91:string)  [unwired: 14 in]
      }
      frame "Data: Initialize" {
        w93 = ""  # AreaNameD
        w94 = T4 {"Current VI Reference"=refnum, "Close Panel on Exit?"=FALSE}  # Core
        w96 = TRUE  # Your Boolean data
        w95 = ""  # Your string data
        # "do not delete - used by framework"
        # "Expand Bundle to add new data elements to shift register data."
        # "Add new data here."
        # "Data names and types of shift register data are defined by this bundle."
        # "Initialize the shift-register data, here.\n(data names are defined by what you wire into the bundle function)"
        n35 = Bundle("Core"=w94, "Your Boolean data"=w96, "Your string data"=w95, "AreaNameD"=w93) -> (w98:T3)  [unwired: 1 in]
        n36 = call <vilib>:"Add State(s) to Queue__JKI_lib_State_Machine.vi"("State(s) in (\"\")"=w100) -> ("States Out"=w99:string)  [unwired: 14 in]
      }
      frame "Data: Cleanup" {
        # "Cleanup any data and references, here.\n(this is called automatically, by the Macro: Exit)"
        n37 = Unbundle By Name(w101) -> ("Core.Current VI Reference"=w104:refnum<vi>)
        n38 = Close Reference(reference=w104, error in (no error)=w103) -> (error out=w102:errorcluster)
        n39 = call <vilib>:"Add State(s) to Queue__JKI_lib_State_Machine.vi"("State(s) in (\"\")"=w106) -> ("States Out"=w105:string)  [unwired: 14 in]
      }
      frame "---------- UI ----------" {
        # "Do not put any code in this frame.\n(It is a separator no-op. You can make a copy of this frame to create a new UI frame)"
        n40 = call <vilib>:"Add State(s) to Queue__JKI_lib_State_Machine.vi"("State(s) in (\"\")"=w110) -> ("States Out"=w109:string)  [unwired: 14 in]
      }
      frame "UI: Initialize" {
        # "Initialize the User Interface, here.\n(this is called automatically, by the Macro: Init)"
        n41 = call <vilib>:"Add State(s) to Queue__JKI_lib_State_Machine.vi"("State(s) in Front (\"\")"="DataBase:LoadAreaName", "State(s) in (\"\")"=w115) -> ("States Out"=w114:string)  [unwired: 13 in]
      }
      frame "UI: Cursor Set" {
        # "Argument"
        # "Set and Unset Cursor Busy.\n(Usage: \"UI: Cursor Set >> Busy|Idle\")"
        n42 = case shown="\"Idle\", 默认" w116 {
          tunnel: w118 -> [w123 w125]
          tunnel: [w122 w124] -> w117
          frame "Idle", Default {
            n43 = call <vilib>:"Unset Busy.vi"("error in (no error)"=w123) -> ("error out"=w122:errorcluster)  [unwired: 10 in]
          }
          frame "Busy" {
            n44 = call <vilib>:"Set Busy.vi"("error in (no error)"=w125) -> ("error out"=w124:errorcluster)  [unwired: 9 in, 1 out]
          }
        }
        n45 = call <vilib>:"Add State(s) to Queue__JKI_lib_State_Machine.vi"("State(s) in (\"\")"=w121) -> ("States Out"=w120:string)  [unwired: 14 in]
      }
      frame "UI: Front Panel State" {
        # "Argument"
        # "Set Front Panel Open or Closed\n(Usage: \"UI: Front Panel State >> Open|Close\")"
        n46 = Unbundle By Name(w128) -> ("Core.Current VI Reference"=w127:refnum<vi>)
        n47 = case shown="\"Open\", 默认" w126 {
          tunnel: w130 -> [w136 w149]
          tunnel: [w138 w150] -> w129
          tunnel: w127 -> [w137 w147]
          frame "Open", Default {
            n48 = property class="VI"(reference=w137, error in=w136) -> (reference out=w134:refnum<vi>, error out=w135:errorcluster, "Front Panel.Open"=w133:bool)
            n49 = case shown="假" w133 {
              tunnel: [w141 w144] -> w138
              tunnel: w135 -> [w140 w144]
              tunnel: w134 -> [w139 _]
              frame False {
                n50 = invoke class="VI" method="FP.Open"(reference=w139, error in=w140, "Activate"=TRUE, "State"=T2."Standard") -> (error out=w141:errorcluster)  [unwired: 1 in, 4 out]
              }
              frame True {
              }
            }
          }
          frame "Close" {
            n51 = property class="VI"(reference=w147, error in=w149) -> (reference out=w146:refnum<vi>, error out=w148:errorcluster, "Front Panel.Open"=w145:bool)
            n52 = case shown="真" w145 {
              tunnel: [w151 w154] -> w150
              tunnel: w148 -> [w151 w153]
              tunnel: w146 -> [_ w152]
              frame False {
              }
              frame True {
                n53 = invoke class="VI" method="FP.Close"(reference=w152, error in=w153) -> (error out=w154:errorcluster)  [unwired: 1 in, 2 out]
              }
            }
          }
        }
        n54 = call <vilib>:"Add State(s) to Queue__JKI_lib_State_Machine.vi"("State(s) in (\"\")"=w132) -> ("States Out"=w131:string)  [unwired: 14 in]
      }
      frame "---------- Macro ----------" {
        # "Do not put any code in this frame.\n(It is a separator no-op. You can make a copy of this frame to create a new Macro frame)"
        n55 = call <vilib>:"Add State(s) to Queue__JKI_lib_State_Machine.vi"("State(s) in (\"\")"=w158) -> ("States Out"=w157:string)  [unwired: 14 in]
      }
      frame "Macro: Initialize" {
        w159 = "Data: Initialize\nInitialize Core Data\nUI: Initialize\nUI: Front Panel State >> Open"  # Data: Initialize Initialize Core Data UI: Initialize UI: Front Panel State >> Open
        # "Initialization Macro\n(This is called once, when the VI starts)"
        n56 = call <vilib>:"Add State(s) to Queue__JKI_lib_State_Machine.vi"("State(s) in Front (\"\")"=w159, "State(s) in (\"\")"=w163) -> ("States Out"=w162:string)  [unwired: 13 in]
      }
      frame "Macro: Exit" {
        # "Exit Macro\n(This is called once, when the VI exits)"
        n57 = Unbundle By Name(w170) -> ("Core.Close Panel on Exit?"=w169:bool)
        n58 = Select(t="UI: Front Panel State >> Close", s=w169, f="") -> (s? t:f=w166:string)
        n59 = call <vilib>:"Add State(s) to Queue__JKI_lib_State_Machine.vi"("State(s) in (\"\")"=w166, "State(s) at Back (\"\")"="Data: Cleanup\nExit") -> ("States Out"=w164:string)  [unwired: 13 in]
        n60 = call <vilib>:"Add State(s) to Queue__JKI_lib_State_Machine.vi"("State(s) in Front (\"\")"=w164, "State(s) in (\"\")"=w173) -> ("States Out"=w172:string)  [unwired: 13 in]
      }
      frame "---------- New Category ----------" {
        # "Template Separator\n(You can make a copy of, or modify, this frame)"
        n61 = call <vilib>:"Add State(s) to Queue__JKI_lib_State_Machine.vi"("State(s) in (\"\")"=w177) -> ("States Out"=w176:string)  [unwired: 14 in]
      }
      frame "New Category: 1" {
        # "Your code here.\n(You can make a copy of, or modify, this frame)"
        n62 = call <vilib>:"Add State(s) to Queue__JKI_lib_State_Machine.vi"("State(s) in (\"\")"=w181) -> ("States Out"=w180:string)  [unwired: 14 in]
      }
      frame "New Category: 2" {
        # "Your code here.\n(You can make a copy of, or modify, this frame)"
        n63 = call <vilib>:"Add State(s) to Queue__JKI_lib_State_Machine.vi"("State(s) in (\"\")"=w185) -> ("States Out"=w184:string)  [unwired: 14 in]
      }
      frame "----------DataBase---------" {
        # "Your code here.\n(You can make a copy of, or modify, this frame)"
        n64 = call <vilib>:"Add State(s) to Queue__JKI_lib_State_Machine.vi"("State(s) in (\"\")"=w189) -> ("States Out"=w188:string)  [unwired: 14 in]
      }
      frame "Database:ImportDecElec" {
        # "Your code here.\n(You can make a copy of, or modify, this frame)"
        n65 = flat-sequence {
          frame #0 {
            n66 = call-poly <vilib>:"Read From Spreadsheet File.vi"("delimiter (\\t)"="," ("delimiter (\\t)"), "file path (dialog if empty)"="导入电极s") -> ("all rows"=w197:string[][])  [unwired: 5 in, 4 out]
            n67 = Array Subset(array=w197, index (row)=1 ("索引 (行)")) -> (w195:string[][])  [unwired: 3 in]
            n68 = for {
              tunnel: w195 -> [w206] mode=indexing
              (unwired) "t_detection_electrodes" ("table")
              n69 = Index Array(array=w206, index=11) -> (element=w200:string)
              n70 = Index Array(array=w206, index=10) -> (element=w201:string)
              n71 = Index Array(array=w206, index=0) -> (element=w215:string)
              n72 = Index Array(array=w206, index=1) -> (element=w214:string)
              n73 = Index Array(array=w206, index=2) -> (element=w213:string)
              n74 = Index Array(array=w206, index=3) -> (element=w212:string)
              n75 = Index Array(array=w206, index=4) -> (element=w211:string)
              n76 = Index Array(array=w206, index=5) -> (element=w210:string)
              n77 = Index Array(array=w206, index=8) -> (element=w207:string)
              n78 = Index Array(array=w206, index=9) -> (element=w202:string)
              n79 = Index Array(array=w206, index=6) -> (element=w209:string)
              n80 = Index Array(array=w206, index=7) -> (element=w208:string)
              n81 = Bundle("String"=w215, "String"=w214, "String"=w213, "String"=w212, "String"=w211, "String"=w210, "String"=w209, "String"=w208, "String"=w207, "String"=w202, "String"=w201, "String"=w200) -> (w199:T5)  [unwired: 1 in]
              n82 = call "InsertDataDE.vi"("检测电极"=w199) -> ()  [unwired: 10 in, 1 out]
              "数组" <- w206
            }
          }
          frame #1 {
            n83 = One Button Dialog(message="电极导入成功") -> ()  [unwired: 1 in, 1 out]
          }
        }
        n84 = call <vilib>:"Add State(s) to Queue__JKI_lib_State_Machine.vi"("State(s) in (\"\")"=w193) -> ("States Out"=w192:string)  [unwired: 14 in]
      }
      frame "DataBase:InsertDecElectrodesInfo" {
        # "Your code here.\n(You can make a copy of, or modify, this frame)"
        n85 = property on="电极管理_新增" class="Tbl (严格)"() -> ("Value"=w230:string[][])  [unwired: 2 in, 2 out]
        n86 = Array Subset(array=w230, index (row)=0 ("索引")) -> (w231:string[][])  [unwired: 3 in]
        n87 = for {
          tunnel: w231 -> [w244] mode=indexing
          tunnel: [w234] -> w227
          tunnel: w228 -> [w235]
          (unwired) "t_detection_electrodes" ("table")
          n88 = local read "区域名称"() -> (w243:u16)
          n89 = property on="区域名称" class="Ring (严格)"() -> ("Strings []"=w242:string[])  [unwired: 2 in, 2 out]
          n90 = Index Array(array=w242, index=w243) -> (element=w241:string)
          n91 = Insert Into Array(array=w244, index=1 ("索引"), new element=w241) -> (w236:string[])
          n92 = Insert Into Array(array=w236, index=0, new element="0" ("新元素/子数组")) -> (w239:string[])
          n93 = Array To Cluster(array=w239) -> ()  [unwired: 1 out]
          n94 = call "InsertDataDE.vi"("error in"=w235) -> ("error out"=w234:errorcluster)  [unwired: 10 in]
        }
        n95 = call <vilib>:"Add State(s) to Queue__JKI_lib_State_Machine.vi"("State(s) in (\"\")"=w233) -> ("States Out"=w232:string)  [unwired: 14 in]
      }
      frame "DataBase:LoadAreaName" {
        # "Your code here.\n(You can make a copy of, or modify, this frame)"
        n96 = local write "电极管理_新增"(string[][] []) -> ()
        n97 = call "SelectData.vi"("SQL query"="select area_name from t_area;", "error in"=w251) -> ("recordset data"=w253:variant[][])  [unwired: 6 in, 1 out]
        n98 = call "ReadDataFromDatabase.vi"("长度"=1, "index"=0, "recordset data"=w253) -> ("所有记录"=w256:string[][])  [unwired: 7 in, 1 out]
        n99 = local read "区域名称"() -> (w248:u16)
        n100 = Index Array(array=w256, index (col)=0 ("索引")) -> (element=w249:string[])  [unwired: 1 in]
        n101 = Index Array(array=w249, index=w248) -> (element=w245:string)
        "AreaName" <- w245
        n102 = property on="区域名称" class="Ring (严格)"("Strings []"=w249) -> ()  [unwired: 2 in, 2 out]
        n103 = Bundle By Name(cluster=w247, "AreaNameD"=w245) -> (w246:T3)
        n104 = call <vilib>:"Add State(s) to Queue__JKI_lib_State_Machine.vi"("State(s) in (\"\")"=w259) -> ("States Out"=w258:string)  [unwired: 14 in]
      }
    }
  }
  n105 = property on="区域名称" class="Ring (严格)" props=["Strings []"]() -> ()  [unwired: 2 in, 3 out]
